vi "Marker Search.vi"(8 "error in (no error)":errorcluster, 9 "Mark Search (0: Highest)":u16(ring) items=["Highest", "Next Peak", "Next Peak Left", "Next Peak Right", "Minimum", "Pk-Pk Search"], 10 "Active Marker (1: Marker1)":u16(ring)=1 items=["Marker1"=1, "Marker2"=2, "Marker3"=3, "Marker4"=4], 11 "VISA resource name":refnum<visa-resource-name>) -> (0 "error out":errorcluster, 3 "VISA resource name out":refnum<visa-resource-name>)   [LabVIEW 2014, in "Agilent ESA PSA Series.lvlib"]
doc: "Specifies the type of marker search and performs the search."
uses:
  Agilent ESA PSA Series.lvlib
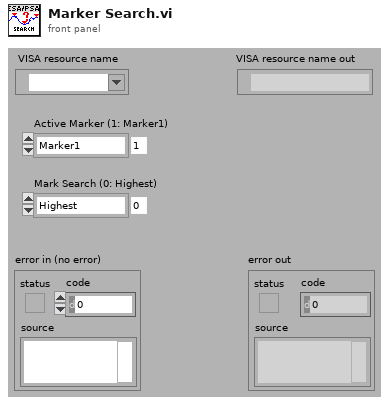
[diagram p1: front panel]
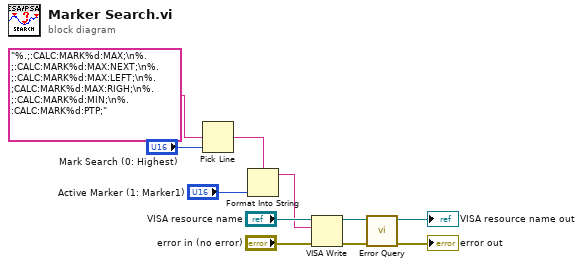
[diagram p0: block diagram]
diagram:
  n1 = Pick Line(multi-line string="%.;:CALC:MARK%d:MAX;\n%.;:CALC:MARK%d:MAX:NEXT;\n%.;:CALC:MARK%d:MAX:LEFT;\n%.;CALC:MARK%d:MAX:RIGH;\n%.;:CALC:MARK%d:MIN;\n%.:CALC:MARK%d:PTP;", line index="Mark Search (0: Highest)") -> (output string=w3:string)  [unwired: 1 in]
  n2 = Format Into String(format string=w3, "Active Marker (1: Marker1)") -> (resulting string=w2:string)  [unwired: 2 in, 1 out]
  n3 = VISA Write(VISA resource name="VISA resource name", write buffer=w2, error in (no error)="error in (no error)") -> (VISA resource name out=w9:refnum<visa-resource-name>, error out=w7:errorcluster)  [unwired: 1 out]
  n4 = call "Error Query.vi"("error in (no error)"=w7, "VISA resource name"=w9) -> ("error out"=→"error out":errorcluster, "VISA resource name out"=→"VISA resource name out":refnum<visa-resource-name>)  [unwired: 6 in, 2 out]
